vi "PH_Beckhoff_StepMot.panel.vi"(0 "object ref":refnum<vi>, 5 "error in (no error)":errorcluster) -> (19 "error out":errorcluster)   [LabVIEW 2014, in "PH_Beckhoff_StepMot.lvlib"]
doc: "This a GUI.\n\nLicense Agreement for this software:\n\nCopyright (C)\nGesellschaft für Schwerionenforschung, GSI\nPlanckstr. 1\n64291 Darmstadt\nGermany\n\nContact: D.Beck@gsi.de \n\nThis program is free software; you can redistribute it and/or modify it under the terms of the GNU General Public License as published by the Free Software Foundation; either version 2 of the license, or (at your option) any later version.\n\nThis program is distributed in the hope that it will be useful, but WITHOUT ANYW ARRANTY; without even the implied warranty of MERCHANTABILITY or FITNESS FOR A PARTICULAR PURPOSE. See the GNU General License for more details (http://www.gnu.org).\n\nGesellschaft für Schwerionenforschung, GSI\nPlanckstr. 1, 64291 Darmstadt, Germany\nFor all questions and ideas contact: M.Richter@gsi.de, H.Brand@gsi.de or D.Beck@gsi.de.\nLast update: 18-DEC-2002"
uses:
  PH_Beckhoff_StepMot.lvlib
  PH_Beckhoff/PH_Beckhoff.Connectivity.ctl
  PH_Beckhoff/PH_Beckhoff.ADS Error.ctl
  PH_Beckhoff/PH_Beckhoff.Values.ctl
  PH_Beckhoff/PH_Beckhoff.Sonderklemmen Inputs.ctl
  PH_Beckhoff/PH_Beckhoff.Analog Inputs.ctl
  PH_Beckhoff/PH_Beckhoff.Scaling Type.ctl
  PH_Beckhoff/PH_Beckhoff.Analog Outputs.ctl
  PH_Beckhoff/PH_Beckhoff.Digital Inputs.ctl
  PH_Beckhoff/PH_Beckhoff.Digital Outputs.ctl
  PH_Beckhoff_StepMot.Axis Cluster.ctl
  non_GPL/instr.lib/Beckhoff/Specials/Step Motor Klemmen/Beckhoff.Step Motor - Motor Configuration.ctl
  non_GPL/instr.lib/Beckhoff/Read and Write Register/Step Motor Klemmen/Beckhoff.Step Motor - Feature Register 1.ctl
  non_GPL/instr.lib/Beckhoff/Read and Write Register/Step Motor Klemmen/Beckhoff.Step Motor - Feature Register 2.ctl
  PH_Stepmotor_BaseClass/PH_Stepmotor_BaseClass.Axis Settings.ctl
  PH_Stepmotor_BaseClass/PH_Stepmotor_BaseClass.Motor Type.ctl
  PH_Stepmotor_BaseClass/PH_Stepmotor_BaseClass.Axis Information.ctl
  PH_Stepmotor_BaseClass/PH_Stepmotor_BaseClass.Axis Activity.ctl
  non_GPL/instr.lib/Beckhoff/Read and Write Data/Step Motor Klemmen/Beckhoff.Step Motor - Status.ctl
  non_GPL/instr.lib/Beckhoff/Read and Write Data/Step Motor Klemmen/Beckhoff.Step Motor - Status Byte.ctl
  non_GPL/instr.lib/Beckhoff/Read and Write Data/Step Motor Klemmen/Beckhoff.Step Motor - Status Word.ctl
  PH_Beckhoff/PH_Beckhoff.GUI Refs.ctl
  PH_Stepmotor_BaseClass/PH_Stepmotor_BaseClass.GUI Refs.ctl
  CSCore/CSObj/CSObj.lvlib
  PH_Common/PH_Common.lvlib
  PH_Beckhoff/PH_Beckhoff.lvlib
  CSCore/CSSystem/CSSystemLib/CSSystemLib.lvlib
  PH_Stepmotor_BaseClass/PH_Stepmotor_BaseClass.lvlib
  PH_Class/PH_Class.lvlib
  non_GPL/instr.lib/Beckhoff/Beckhoff - Driver np.lvlib
panel:
  in  "Tab Control":enum32{"Beckhoff Stuff", "Stepper Motors"}(tab)=enum."Stepper Motors"
  out "Current Values":T1
  in  "Show Info":bool
  out "configured?":bool
  out "Prdc Int [ms]":i32
  out "Connection":T8
  out "IP":string
  out "ADS Error":T9
  in  "Get Settings":bool
  out "Axes Settings (Beckhoff Class)":T10[](array[typedef])
  out "Axes PSDB Infos":T14(array[cluster])
  out "Axes Configuration (Base Class)":T19(array[cluster])
  out "Stati":T20[](array[typedef])
  in  "Delete":bool
  in  "Exit":bool
  # "PCS"
  # "3.40"
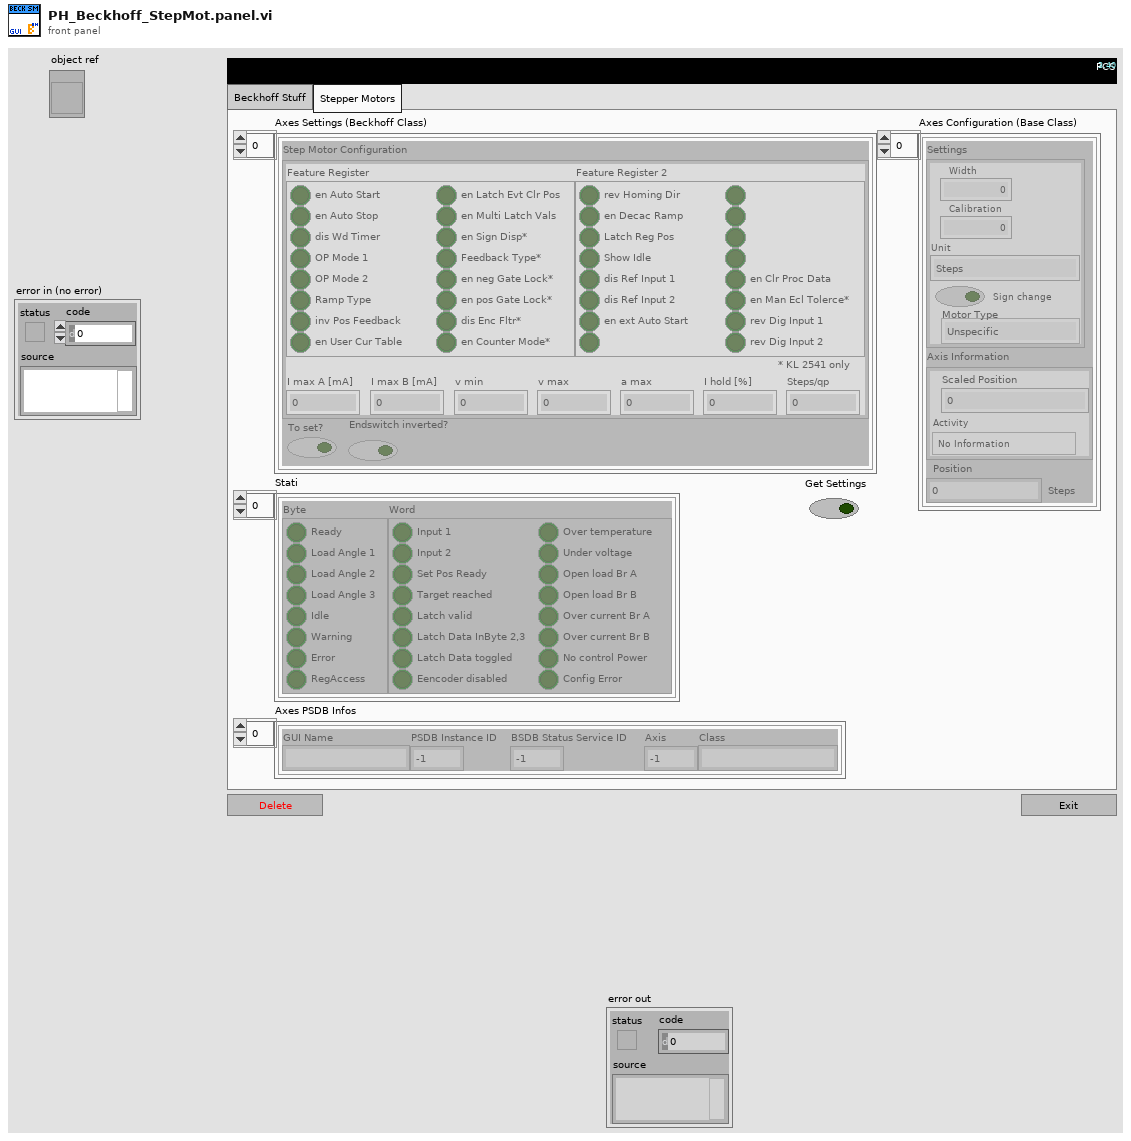
[diagram p1: front panel]
types:
  T1 = typedef "PH_Beckhoff.lvlib/PH_Beckhoff.Values.ctl" = cluster{"Sonderklemmen Inputs":T2, "Analog Inputs":T3, "Analog Outputs":T5, "Digital Inputs":T6, "Digital Outputs":T7}
  T2 = typedef "PH_Beckhoff.lvlib/PH_Beckhoff.Sonderklemmen Inputs.ctl" = cluster{"Total Length":u32, "Name":string, "Value":u64, "Quality":bool, "Service ID":i32, "Offset":u32, "Length":u32}[]
  T3 = typedef "PH_Beckhoff.lvlib/PH_Beckhoff.Analog Inputs.ctl" = cluster{"Name":string, "Value":u32, "Quality":bool, "Service ID":i32, "Sca Type":T4}[]
  T4 = typedef "PH_Beckhoff.lvlib/PH_Beckhoff.Scaling Type.ctl" = enum16{"none", "0 ... 15 Bit -> 0 ... 5", "0 ... 15 Bit -> 0 ... 10", "0 ... 15 Bit -> 0 ... 25", "0 ... 15 Bit -> 4 ... 20", "0 ... 15 Bit -> 0 ... 1", "0 ... 15 Bit -> 0 ... 20000", "0 ... 15 Bit -> 0 ... 24000"}
  T5 = typedef "PH_Beckhoff.lvlib/PH_Beckhoff.Analog Outputs.ctl" = cluster{"Name":string, "Value":u32, "Quality":bool, "Wanted Value":u32, "Service ID":i32, "Sca Type":T4}[]
  T6 = typedef "PH_Beckhoff.lvlib/PH_Beckhoff.Digital Inputs.ctl" = cluster{"Name":string, "Value":bool, "Quality":bool, "Service ID":i32, "inverted?":bool}[]
  T7 = typedef "PH_Beckhoff.lvlib/PH_Beckhoff.Digital Outputs.ctl" = cluster{"Name":string, "Value":bool, "Quality":bool, "Wanted Value":bool, "Service ID":i32, "inverted?":bool}[]
  T8 = typedef "PH_Beckhoff.lvlib/PH_Beckhoff.Connectivity.ctl" = cluster{"DLL?":bool, "Port?":bool, "Client?":bool, "Ping?":bool, "unsuccessful Pings":u32}
  T9 = typedef "PH_Beckhoff.lvlib/PH_Beckhoff.ADS Error.ctl" = cluster{"Latest Error":string, "Error List":string[]}
  T10 = typedef "PH_Beckhoff_StepMot.lvlib/PH_Beckhoff_StepMot.Axis Cluster.ctl" = cluster{"Step Motor Configuration":T11, "To set?":bool, "Endswitch inverted?":bool}
  T11 = typedef "Beckhoff - Driver np.lvlib/Beckhoff.Step Motor - Motor Configuration.ctl" = cluster{"Feature Register":T12, "I max A [mA]":dbl, "I max B [mA]":dbl, "v min":u32, "v max":u32, "a max":u32, "I hold [%]":u32, "Steps/qp":u32, "Feature Register 2":T13}
  T12 = typedef "Beckhoff - Driver np.lvlib/Beckhoff.Step Motor - Feature Register 1.ctl" = cluster{"en Auto Start":bool, "en Auto Stop":bool, "dis Wd Timer":bool, "OP Mode 1":bool, "OP Mode 2":bool, "Ramp Type":bool, "inv Pos Feedback":bool, "en User Cur Table":bool, "en Latch Evt Clr Pos":bool, "en Multi Latch Vals":bool, "en Sign Disp*":bool, "Feedback Type*":bool, "en neg Gate Lock*":bool, "en pos Gate Lock*":bool, "dis Enc Fltr*":bool, "en Counter Mode*":bool}
  T13 = typedef "Beckhoff - Driver np.lvlib/Beckhoff.Step Motor - Feature Register 2.ctl" = cluster{"rev Homing Dir":bool, "en Decac Ramp":bool, "Latch Reg Pos":bool, "Show Idle":bool, "dis Ref Input 1":bool, "dis Ref Input 2":bool, "en ext Auto Start":bool, "N/A":bool, "N/A":bool, "N/A":bool, "N/A":bool, "N/A":bool, "en Clr Proc Data":bool, "en Man Ecl Tolerce*":bool, "rev Dig Input 1":bool, "rev Dig Input 2":bool}
  T14 = cluster{"GUI Name":string, "PSDB Instance ID":i32, "BSDB Status Service ID":i32, "Axis":i32, "Class":string}[]
  T15 = typedef "PH_Stepmotor_BaseClass.lvlib/PH_Stepmotor_BaseClass.Axis Settings.ctl" = cluster{"Sign change":bool, "Width":dbl, "Calibration":dbl, "Unit":string, "Motor Type":T16, "Unit Width":string, "Unit CF":string}
  T16 = typedef "PH_Stepmotor_BaseClass.lvlib/PH_Stepmotor_BaseClass.Motor Type.ctl" = enum16{"Unspecific", "OWIS 49.120.2633", "OWIS 49.060.1033", "OWIS 43.040.2558", "Diamond Motion 2200 series", "OWIS 49.120.266B.MV6", "Calorimeter", "Linear Stage 1", "MICOS VT-80", "MICOS VT-80 S", "Standa Rotstage nt0.95A", "PUF RA 320.200", "PUF RA 800.200", "PUF RA 800.400", "PUF RA 400.50", "1324.nn.800.50", "1324.n9c.800.50", "1324.nn.320.200", "1324.nn.400.200", "1324.nn.800.200", "1324.nn.400.50", "1324.8c9c.800.50", "1324.8c9c.400.200"}
  T17 = typedef "PH_Stepmotor_BaseClass.lvlib/PH_Stepmotor_BaseClass.Axis Information.ctl" = cluster{"Scaled Position":dbl, "Activity":T18}
  T18 = typedef "PH_Stepmotor_BaseClass.lvlib/PH_Stepmotor_BaseClass.Axis Activity.ctl" = enum16{"No Information", "stopped", "running", "Failure", "Alarm", "stopped at backward ES", "stopped at foreward ES"}
  T19 = cluster{"Settings":T15, "Axis Information":T17, "Position":i32}[]
  T20 = typedef "Beckhoff - Driver np.lvlib/Beckhoff.Step Motor - Status.ctl" = cluster{"Byte":T21, "Word":T22}
  T21 = typedef "Beckhoff - Driver np.lvlib/Beckhoff.Step Motor - Status Byte.ctl" = cluster{"Ready":bool, "Load Angle 1":bool, "Load Angle 2":bool, "Load Angle 3":bool, "Idle":bool, "Warning":bool, "Error":bool, "RegAccess":bool}
  T22 = typedef "Beckhoff - Driver np.lvlib/Beckhoff.Step Motor - Status Word.ctl" = cluster{"Input 1":bool, "Input 2":bool, "Set Pos Ready":bool, "Target reached":bool, "Latch valid":bool, "Latch Data InByte 2,3":bool, "Latch Data toggled":bool, "Eencoder disabled":bool, "Over temperature":bool, "Under voltage":bool, "Open load Br A":bool, "Open load Br B":bool, "Over current Br A":bool, "Over current Br B":bool, "No control Power":bool, "Config Error":bool}
  T23 = typedef "PH_Stepmotor_BaseClass.lvlib/PH_Stepmotor_BaseClass.GUI Refs.ctl" = cluster{"Axes Configuration":refnum<vi>, "Device Error":refnum<vi>, "Axes PSDB Infos":refnum<vi>}
  T24 = cluster{"Stepmotor Base Class ":T23, "PSDB Status":refnum<vi>}
  T25 = typedef "PH_Beckhoff.lvlib/PH_Beckhoff.GUI Refs.ctl" = cluster{"ADS Error":refnum<vi>, "Values":refnum<vi>, "configured?":refnum<vi>, "Connection":refnum<vi>, "IP":refnum<vi>, "Prdc Int [ms]":refnum<vi>}
  T26 = typedef "PH_Beckhoff.lvlib/PH_Beckhoff.i attribute.ctl" = cluster{"GUI Refs":T25, "operation?":bool, "Default Prdc Interval":i32, "Connection":T8, "AMS Net ID":T27, "Klemmencluster: # of":T28, "Values":T1, "IP":string, "Description":string, "configured?":bool, "Change Manager":cluster{"Detemination wanted?":bool, "Values changed at":cluster{"Sonderklemmen Inputs":i32[], "Analog Inputs":i32[], "Analog Outputs":i32[], "Digital Inputs":i32[], "Digital Outputs":i32[]}}, "Difference to handle an analog input as change":u32}
  T27 = typedef "Beckhoff - Driver np.lvlib/Beckhoff Access.ctl" = cluster{"DLL path":path, "AMS Net ID":cluster{"1st # of IP":u8, "2nd # of IP":u8, "3rd # of IP":u8, "4th # of IP":u8, "In Port":u8, "Out Port":u8}}
  T28 = typedef "Beckhoff - Driver np.lvlib/Klemmendeclarer.ctl" = cluster{"Offset due to Sonderklemms":u32, "analog Inputs":u32, "analog Outputs":u32, "digital Input Bits":u32, "digital Output Bits":u32}
  T29 = typedef "PH_Beckhoff_StepMot.lvlib/PH_Beckhoff_StepMot.i attribute.ctl" = cluster{"Axes Settings":T10[], "GUI Refs":cluster{"Axes Settings":refnum<vi>, "Stati":refnum<vi>}, "Get Beckhoff Settings":bool}
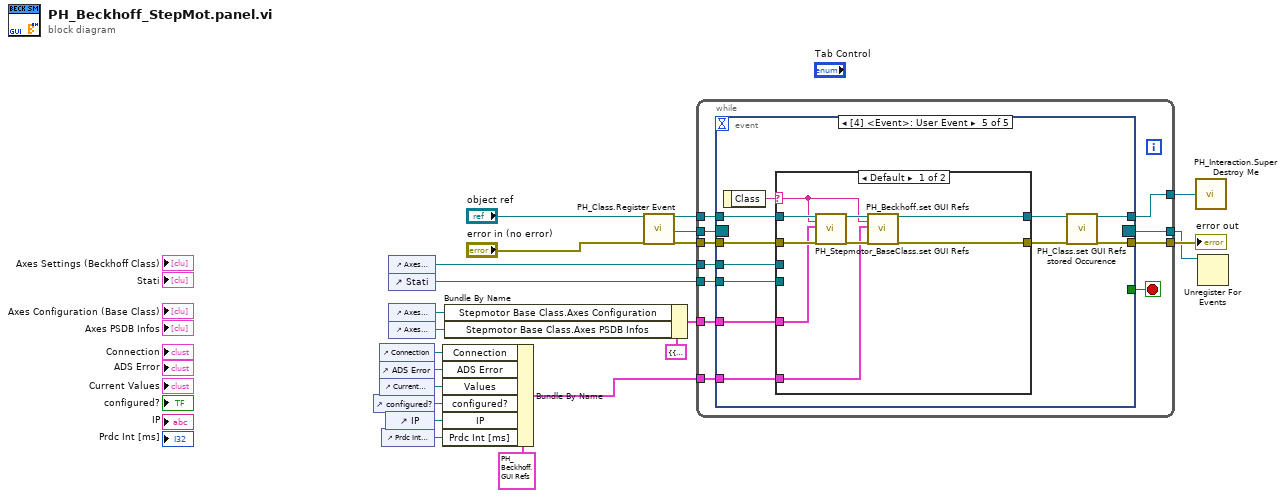
[diagram p0: block diagram]
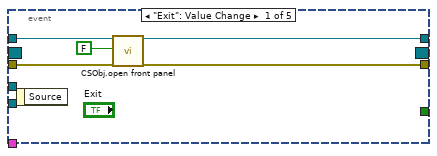
[diagram p2: hidden frame]
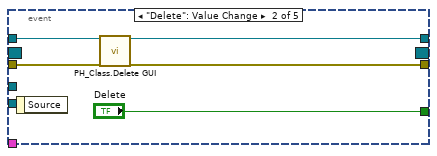
[diagram p3: hidden frame]
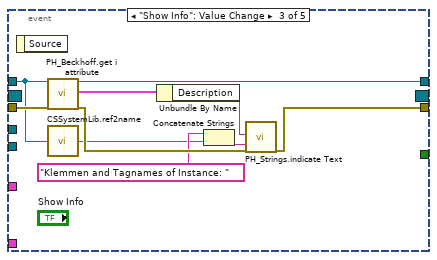
[diagram p4: hidden frame]
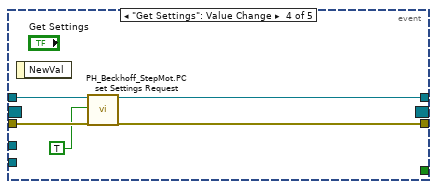
[diagram p5: hidden frame]
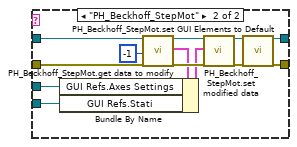
[diagram p6: hidden frame]
diagram:
  n1 = control-ref of="configured?"() -> (w17:refnum<vi>)
  n2 = control-ref of="Connection"() -> (w20:refnum<vi>)
  n3 = control-ref of="ADS Error"() -> (w19:refnum<vi>)
  n4 = control-ref of="Current Values"() -> (w18:refnum<vi>)
  n5 = control-ref of="Prdc Int [ms]"() -> (w2:refnum<vi>)
  n6 = control-ref of="IP"() -> (w3:refnum<vi>)
  n7 = control-ref of="Axes Settings (Beckhoff Class)"() -> (w10:refnum<vi>)
  n8 = control-ref of="Stati"() -> (w9:refnum<vi>)
  n9 = control-ref of="Axes Configuration (Base Class)"() -> (w1:refnum<vi>)
  n10 = control-ref of="Axes PSDB Infos"() -> (w15:refnum<vi>)
  n11 = Bundle By Name(cluster=T25 {"ADS Error"=refnum, "Values"=refnum, "configured?"=refnum, "Connection"=refnum, "IP"=refnum, "Prdc Int [ms]"=refnum} ("GUI Dummy"), "Connection"=w20, "ADS Error"=w19, "Values"=w18, "configured?"=w17, "IP"=w3, "Prdc Int [ms]"=w2) -> (w6:T25)
  n12 = Bundle By Name(cluster=T24 {"Stepmotor Base Class "={"Axes Configuration"=refnum, "Device Error"=refnum, "Axes PSDB Infos"=refnum}, "PSDB Status"=refnum} ("GUI Refs"), "Stepmotor Base Class.Axes Configuration"=w1, "Stepmotor Base Class.Axes PSDB Infos"=w15) -> (w8:T24)
  n13 = call "PH_Class.Register Event.vi"("i ref in"="object ref", "error in (no error)"="error in (no error)") -> ("i ref out"=w14:refnum<vi>, "Event Registration Refnum"=w12:refnum<event-registration>, "error out"=w13:errorcluster)  [unwired: 15 in]
  n14 = while {
    tunnel: w14 -> [w30]
    tunnel: [w29] -> w22
    tunnel: w13 -> [w32]
    tunnel: [w31] -> w21
    tunnel: w12 -> [w28]
    tunnel: [w27] -> w11
    tunnel: w10 -> [w26]
    tunnel: w9 -> [w25]
    tunnel: w8 -> [w24]
    tunnel: w6 -> [w23]
    stop <- w33 stop-if-true
    n15 = event shown="[4] <Event>: User Event" {
      selector: w28 -> [_ _ _ _ _]
      dyn-events: [_ _ _ _ _] -> w27
      timeout: _ -> [_ _ _ _ _]
      tunnel: [_ "Delete" _ _ _] -> w33
      tunnel: w30 -> [w35 w40 w44 w58 w68]
      tunnel: w32 -> [w38 w42 w53 w56 w67]
      tunnel: [w37 w41 w50 w55 w62] -> w31
      tunnel: [w34 w39 w52 w57 w59] -> w29
      tunnel: w26 -> [_ _ _ _ w66]
      tunnel: w25 -> [_ _ _ _ w65]
      tunnel: w24 -> [_ _ _ _ w64]
      tunnel: w23 -> [_ _ _ _ w63]
      event "Exit": Value Change {
        n16 = event-data() -> ()  [unwired: 1 in, 1 out]
        n17 = call "CSObj.open front panel.vi"("i ref in"=w35, "frontPanelOpen"=FALSE ("front panel open"), "error in (no error)"=w38) -> ("i ref out"=w34:refnum<vi>, "error out"=w37:errorcluster)  [unwired: 15 in]
      }
      event "Delete": Value Change {
        n18 = event-data() -> ()  [unwired: 1 in, 1 out]
        n19 = call "PH_Class.Delete GUI.vi"("VI in"=w40, "error in (no error)"=w42) -> ("VI out"=w39:refnum<vi>, "error out"=w41:errorcluster)  [unwired: 16 in]
      }
      event "Show Info": Value Change {
        n20 = event-data() -> ()  [unwired: 1 in, 1 out]
        n21 = call "PH_Beckhoff.get i attribute.vi"("i ref in"=w44, "error in (no error)"=w53) -> ("i ref out"=w52:refnum<vi>, "i attribute"=w49:T26, "error out"=w51:errorcluster)  [unwired: 15 in]
        n22 = call "CSSystemLib.ref2name.vi"("obj refnum"=w44) -> ("name"=w45:string)
        n23 = Unbundle By Name(w49) -> ("Description"=w48:string)
        n24 = Concatenate Strings("Klemmen and Tagnames of Instance: " ("Caption.Text"), w45) -> (w46:string)
        n25 = call "PH_Strings.indicate Text.vi"("String to show"=w48, "Caption.Text"=w46, "error in (no error)"=w51) -> ("error out"=w50:errorcluster)  [unwired: 16 in]
      }
      event "Get Settings": Value Change {
        n26 = event-data() -> ()  [unwired: 1 in, 1 out]
        n27 = call "PH_Beckhoff_StepMot.PC set Settings Request.vi"("VI in"=w58, "Get Beckhoff Settings"=TRUE ("Get Beckhoff Config"), "error in (no error)"=w56) -> ("VI out"=w57:refnum<vi>, "error out"=w55:errorcluster)  [unwired: 15 in]
      }
      event User Event {
        n28 = event-data() -> ("Class"=w69:string)  [unwired: 1 in]
        n29 = case shown="Default" w69 {
          selector: w69 -> [w70 _]
          tunnel: w68 -> [w78 w86]
          tunnel: [w74 w80] -> w60
          tunnel: w67 -> [w77 w85]
          tunnel: [w72 w79] -> w61
          tunnel: w66 -> [_ w84]
          tunnel: w65 -> [_ w83]
          tunnel: w64 -> [w76 _]
          tunnel: w63 -> [w71 _]
          frame Default {
            n30 = call "PH_Stepmotor_BaseClass.set GUI Refs.vi"("i ref in"=w78, "Class"=w70, "GUI Refs"=w76, "error in"=w77) -> ("i ref out"=w75:refnum<vi>, "error out"=w73:errorcluster)  [unwired: 14 in]
            n31 = call "PH_Beckhoff.set GUI Refs.vi"("i ref in"=w75, "Class"=w70, "GUI Refs"=w71, "error in"=w73) -> ("i ref out"=w74:refnum<vi>, "error out"=w72:errorcluster)  [unwired: 14 in]
          }
          frame "PH_Beckhoff_StepMot" {
            n32 = call "PH_Beckhoff_StepMot.get data to modify.vi"("i ref in"=w86, "ms timeout (10000)"=-1, "error in (no error)"=w85) -> ("i ref out"=w89:refnum<vi>, "i attribute"=w88:T29, "error out"=w91:errorcluster)  [unwired: 13 in, 1 out]
            n33 = Bundle By Name(cluster=w88, "GUI Refs.Axes Settings"=w84, "GUI Refs.Stati"=w83) -> (w87:T29)
            n34 = call "PH_Beckhoff_StepMot.set modified data.vi"("i ref in"=w89, "i attribute"=w87, "error in (no error)"=w91) -> ("i ref out"=w82:refnum<vi>, "error out"=w81:errorcluster)  [unwired: 15 in]
            n35 = call "PH_Beckhoff_StepMot.set GUI Elements to Default.vi"("i ref in"=w82, "error in"=w81) -> ("i ref out"=w80:refnum<vi>, "error out"=w79:errorcluster)  [unwired: 16 in]
          }
        }
        n36 = call "PH_Class.set GUI Refs stored Occurence.vi"("i ref in"=w60, "error in (no error)"=w61) -> ("i ref out"=w59:refnum<vi>, "error out"=w62:errorcluster)  [unwired: 16 in]
      }
    }
  }
  "error out" <- w21
  n37 = call "PH_Interaction.Super Destroy Me.vi"("i ref out"=w22) -> ()
  n38 = Unregister For Events(event registration refnum=w11) -> ()  [unwired: 1 in, 1 out]
